vi "TL add waypoints.vi"(2 "error in":errorcluster, 3 "MDF":T1(array[cluster]), 4 "Image In":T2) -> (0 "error out":errorcluster, 1 "Image Out":T2)   [LabVIEW 2014]
doc: "This vi will overlay the waypoints created in the Mission Definition File onto the pool image."
uses:
  <vilib>/vision/Image Controls.llb/IMAQ Image.ctl
panel:
  out "size(s)":i32
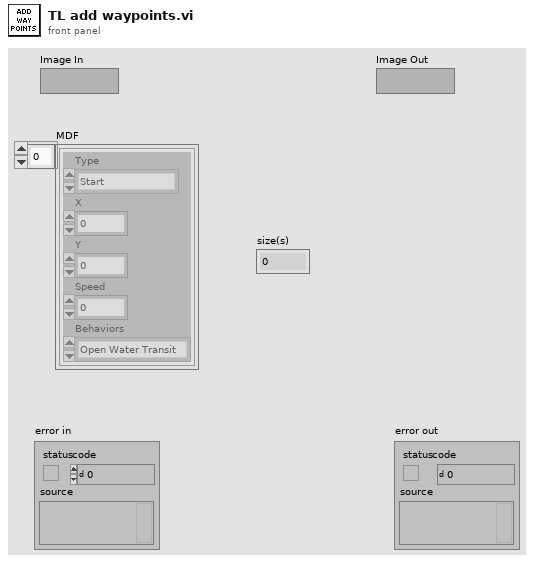
[diagram p1: front panel]
types:
  T1 = cluster{"Type":enum16{"Start", "Buoy Circling", "Waypoint", "End"}, "X":i32, "Y":i32, "Speed":i32, "Behaviors":enum16{"Open Water Transit", "P-Wall Follow", "S-Wall Follow", "Get Unstuck"}}[]
  T2 = typedef "IMAQ Image.ctl" = refnum<image>
  T3 = enum16{"Start", "Buoy Circling", "Waypoint", "End"}
  T4 = cluster{"Type":enum16{"Start", "Buoy Circling", "Waypoint", "End"}, "X":i32, "Y":i32, "Speed":i32, "Behaviors":enum16{"Open Water Transit", "P-Wall Follow", "S-Wall Follow", "Get Unstuck"}}
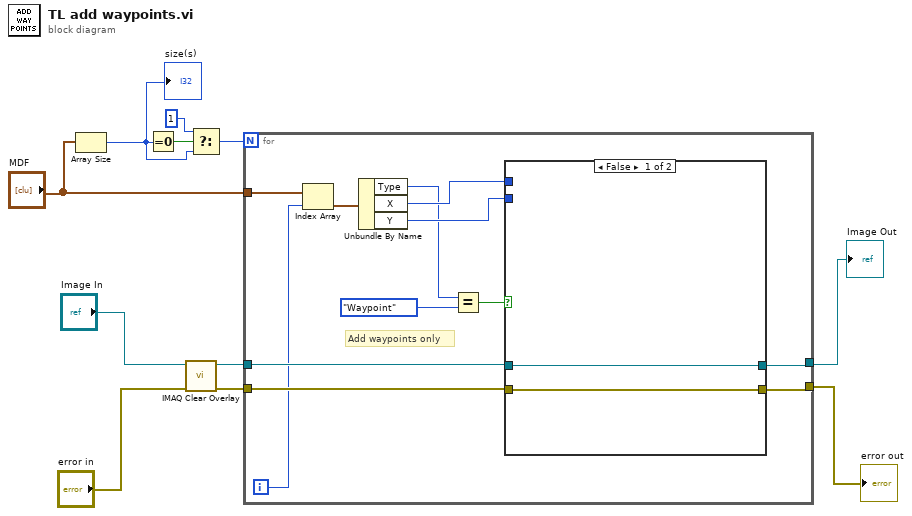
[diagram p0: block diagram]
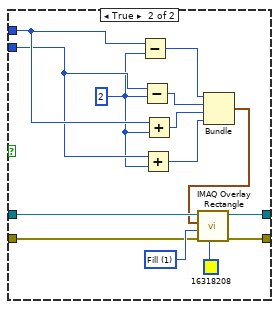
[diagram p2: hidden frame]
diagram:
  n1 = Array Size(array="MDF") -> (size(s)=w1:i32)
  "size(s)" <- w1
  n2 = Equal To 0?(x=w1) -> (x = 0?=w4:bool)
  n3 = call "IMAQ Clear Overlay"("error in (no error)"="error in", "Image"="Image In") -> ("error out"=w8:errorcluster, "Image Out"=w6:T2)  [unwired: 8 in]
  n4 = Select(t=1, s=w4, f=w1) -> (s? t:f=w2:i32)
  n5 = for {
    N: w2 -> [_]
    tunnel: [w23] -> w11
    tunnel: [w22] -> w10
    tunnel: w8 -> [w21]
    tunnel: w6 -> [w20]
    tunnel: "MDF" -> [w19]
    i -> [w18]
    # "Add waypoints only"
    n6 = Index Array(array=w19, index=w18) -> (element=w17:T4)
    n7 = Unbundle By Name(w17) -> ("Type"=w13:T3, "X"=w16:i32, "Y"=w15:i32)
    n8 = Equal?(x=w13, y=T3."Waypoint" ("Type")) -> (x = y?=w14:bool)
    n9 = case shown="False" w14 {
      tunnel: [w25 w37] -> w23
      tunnel: [w24 w36] -> w22
      tunnel: w21 -> [w24 w35]
      tunnel: w20 -> [w25 w34]
      tunnel: w16 -> [_ w33]
      tunnel: w15 -> [_ w32]
      frame False {
      }
      frame True {
        w31 = 2
        w38 = u32 1 items=["Frame", "Fill", "Highlight"] ("Drawing Mode (Frame)")
        n10 = Subtract(x=w33, y=w31) -> (x-y=w30:i32)
        n11 = Subtract(x=w32, y=w31) -> (x-y=w29:i32)
        n12 = Add(x=w32, y=w31) -> (x+y=w27:i32)
        n13 = Add(x=w33, y=w31) -> (x+y=w28:i32)
        n14 = Bundle(w30, w29, w28, w27) -> (w26:cluster{i32, i32, i32, i32})  [unwired: 1 in]
        n15 = call "IMAQ Overlay Rectangle"("Color"=u32 16318208, "error in (no error)"=w35, "Drawing Mode (Frame)"=w38, "Rectangle"=w26, "Image"=w34) -> ("error out"=w36:errorcluster, "Image Out"=w37:T2)  [unwired: 5 in]
      }
    }
  }
  "Image Out" <- w11
  "error out" <- w10
